vi "initializeHeartbeat.vi"(8 "error in (no error)":errorcluster, 11 "MonoClientCommunicator in":refnum<class "MonoClientCommunicator.lvclass">) -> (0 "error out":errorcluster, 3 "MonoClientCommunicator out":refnum<class "MonoClientCommunicator.lvclass">)   [LabVIEW 2016, in "MonoClientCommunicator.lvclass"]
uses:
  MonoClientCommunicator.lvclass
  MonoClientCommunicator.lvclass/MonoClientCommunicator.ctl
  MonoHeartbeat/MonoHeartbeat.lvclass
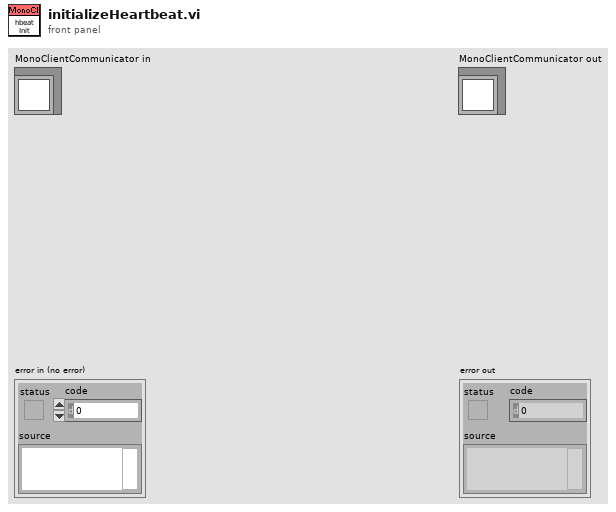
[diagram p1: front panel]
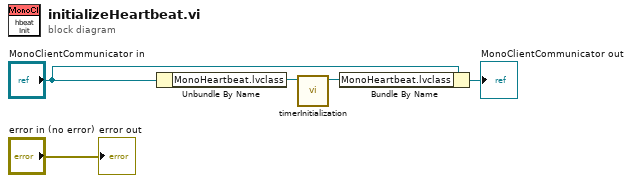
[diagram p0: block diagram]
diagram:
  n1 = Unbundle By Name("MonoClientCommunicator in") -> ("MonoHeartbeat.lvclass"=w4:refnum<class "MonoHeartbeat.lvclass">)
  n2 = call "timerInitialization.vi"("MonoHeartbeat in"=w4) -> ("MonoHeartbeat out"=w2:refnum<class "MonoHeartbeat.lvclass">)  [unwired: 9 in, 1 out]
  n3 = Bundle By Name(cluster="MonoClientCommunicator in", "MonoHeartbeat.lvclass"=w2) -> (→"MonoClientCommunicator out":refnum<class "MonoClientCommunicator.lvclass">)
  "error out" <- "error in (no error)"
